vi "ADI_IMU_ADIS16470_WriteReadRegister.vi"(8 "error in (no error)":errorcluster, 9 "Data":u16=2049, 10 "Register":T1=54 items=["SMPL_PRD"=54, "SENS_AVG"=56, "MSC_CTRL"=52, "ERROR_FLAGS"=60, "TEMP"=44, "BARO"=40, "Z_MAG"=36, "Y_MAG"=32, "X_MAG"=28, "Z_ACCEL"=24, "Y_ACCEL"=20, "X_ACCEL"=16, "Z_GYRO"=12, "Y_GYRO"=8, "X_GYRO"=4, "PID"=86], 11 "SPIDevRef in":T2) -> (0 "error out":errorcluster, 1 "Write OK?":bool, 2 "Register Value":u16, 3 "SPIDevRef out":T2)   [LabVIEW 2017, in "ADIS16470_IMU.lvlib"]
uses:
  ADIS16470_IMU.lvlib
  <vilib>/Rock Robotics/WPI/SPI/WPI_SPIDevRef.ctl
  <vilib>/Rock Robotics/SystemInterfaces/spilib/spi_bus.ctl
  ADI_IMU_ADIS16470_Registers.ctl
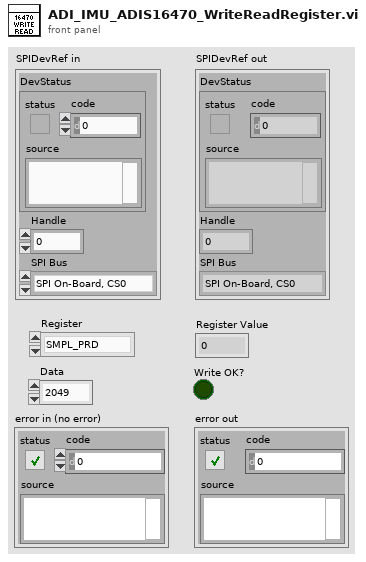
[diagram p1: front panel]
types:
  T1 = typedef "ADIS16470_IMU.lvlib/ADI_IMU_ADIS16470_Registers.ctl" = u8
  T2 = typedef "WPI_SPIDevRef.ctl" = cluster{"DevStatus":errorcluster, "Handle":i32, "SPI Bus":T3}
  T3 = typedef "spi_bus.ctl" = enum16{"SPI On-Board, CS0", "SPI On-Board, CS1", "SPI On-Board, CS2", "SPI On-Board, CS3", "SPI MXP", "Invalid"}
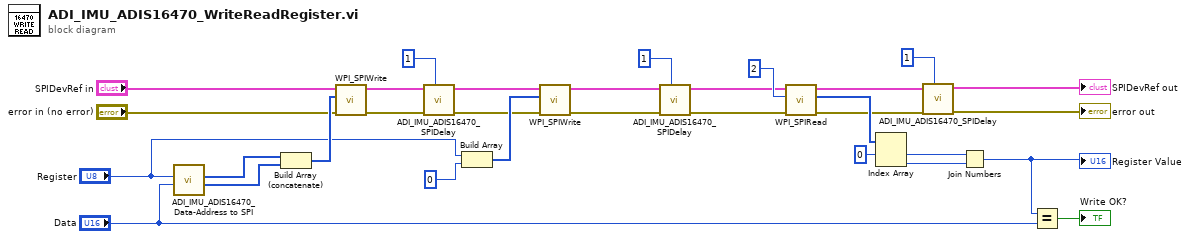
[diagram p0: block diagram]
diagram:
  n1 = call "ADI_IMU_ADIS16470_Data-Address to SPI.vi"("Data"="Data", "Address"="Register") -> ("High Word"=w26:u8[], "Low Word"=w27:u8[])  [unwired: 8 in]
  n2 = Build Array (concatenate)(w27, w26) -> (w28:u8[])
  n3 = call <vilib>:"WPI_SPIWrite.vi"("error in (no error)"="error in (no error)", "Data To Send"=w28, "SPIDevRef"="SPIDevRef in") -> ("error out"=w12:errorcluster, "SPIDevRef"=w13:T2)  [unwired: 7 out]
  n4 = call "ADI_IMU_ADIS16470_SPIDelay.vi"("Wait (ms)"=u32 1, "error in"=w12, "SPIDevRef in"=w13) -> ("error out"=w14:errorcluster, "SPIDevRef out"=w15:T2)  [unwired: 7 in]
  n5 = Build Array("Register", 0) -> (w25:i32[])
  n6 = call <vilib>:"WPI_SPIWrite.vi"("error in (no error)"=w14, "Data To Send"=w25, "SPIDevRef"=w15) -> ("error out"=w10:errorcluster, "SPIDevRef"=w11:T2)  [unwired: 7 out]
  n7 = call "ADI_IMU_ADIS16470_SPIDelay.vi"("Wait (ms)"=u32 1, "error in"=w10, "SPIDevRef in"=w11) -> ("error out"=w9:errorcluster, "SPIDevRef out"=w8:T2)  [unwired: 7 in]
  n8 = call <vilib>:"WPI_SPIRead.vi"("error in (no error)"=w9, "Num to Read"=2, "SPIDevRef"=w8) -> ("error out"=w6:errorcluster, "Received Data"=w29:u8[], "SPIDevRef"=w7:T2)  [unwired: 6 in]
  n9 = Index Array(array=w29, index #1=0 ("index")) -> (element #1=w22:u8, element #2=w21:u8)  [unwired: 1 in]
  n10 = call "ADI_IMU_ADIS16470_SPIDelay.vi"("Wait (ms)"=u32 1, "error in"=w6, "SPIDevRef in"=w7) -> ("error out"=→"error out":errorcluster, "SPIDevRef out"=→"SPIDevRef out":T2)  [unwired: 7 in]
  n11 = Join Numbers(hi=w22, lo=w21) -> ((hi.lo)=w20:u16)
  "Register Value" <- w20
  n12 = Equal?(x=w20, y="Data") -> (x = y?=→"Write OK?":bool)
